vi "DAQ_DC-RMS Voltage Meas Initialize.vi"(0 "Physical Channels":tag, 7 "Global Channels":refnum<k21>, 11 "error in":errorcluster) -> (4 "DAQmx Task Out":refnum<k21>, 15 "error out":errorcluster)   [LabVIEW 2021, in "DAQ_DC-RMS Voltage Measurement.lvlib"]
doc: "Initialize analog input channels and obtains a DAQmx task\n\nProvide either Physical channel or Global Channel\nIf both physical and Global channels are provided, Global Channels will take precedence"
uses:
  DAQ_DC-RMS Voltage Measurement.lvlib
  <vilib>/DAQmx/create/channels.llb/DAQmx Create Channel (AI-Voltage-Basic).vi
panel:
  # "Inputs"
  # "Outputs"
  # "Overview:\nThis VI interacts with the DAQ driver to initialize an instrument and provide a corresponding instrument handle\n\nHardware Requirements: A compatible PXI, PCIe, USB, cDAQ or Testscale device\n\nSoftware Requirements: NI DAQmx 2022 Q4 or later\n\nInstructions:\n1. Enter physical channel in which DC Voltage Measurement has to be done in Physical Channels control. (Or) Enter Global channels to use it instead of initiating a new task. User must configure only one input. If both are provided, Global Channels will take precedence.\n3. Get the DC Voltage Measurement task from DAQmx Task Out\n\nNote: User can use the DAQmx Task on other APIs to configure and initiate DC-RMS Voltage and Measurements."
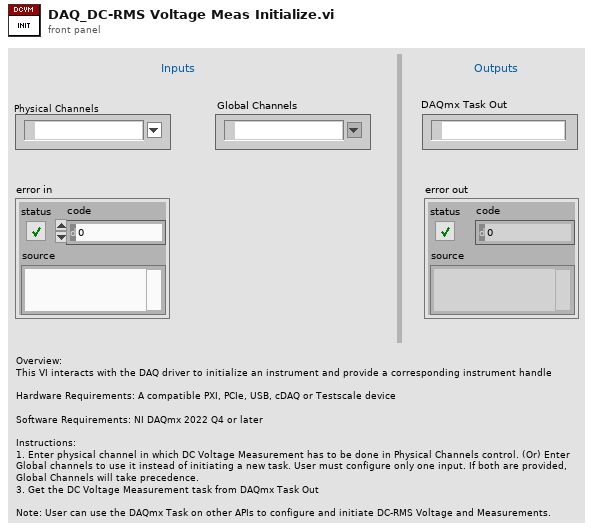
[diagram p1: front panel]
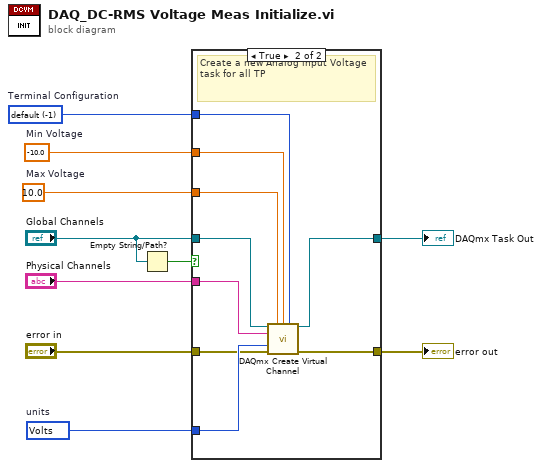
[diagram p0: block diagram]
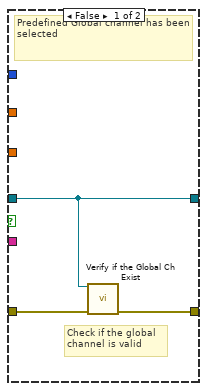
[diagram p2: hidden frame]
diagram:
  w3 = -1 items=["default"=-1, "RSE"=10083, "NRSE"=10078, "Differential"=10106, "Pseudodifferential"=12529]  # Terminal Configuration
  w4 = -10.0  # Min Voltage
  w5 = 10.0  # Max Voltage
  w10 = 10348 items=["Volts"=10348, "From Custom Scale"=10065]  # units
  n1 = Empty String/Path?(string/path="Global Channels") -> (empty?=w2:bool)
  n2 = case shown="True" w2 {
    tunnel: "Physical Channels" -> [_ w18]
    tunnel: "Global Channels" -> [w11 w22]
    tunnel: [w11 w21] -> w6
    tunnel: "error in" -> [w13 w19]
    tunnel: [w12 w17] -> w9
    tunnel: w10 -> [_ w20]
    tunnel: w5 -> [_ w16]
    tunnel: w4 -> [_ w15]
    tunnel: w3 -> [_ w14]
    frame False {
      # "Check if the global\nchannel is valid"
      # "Predefined Global channel has been selected"
      n3 = call "Verify if the Global Ch Exist.vi"("Global Channels"=w11, "error in (no error)"=w13) -> ("error out"=w12:errorcluster)  [unwired: 13 in]
    }
    frame True {
      # "Create a new Analog input Voltage task for all TP"
      n4 = call-poly <vilib>:"DAQmx Create Virtual Channel.vi"("task in"=w22, "maximum value"=w16, "minimum value"=w15, "input terminal configuration"=w14, "physical channels"=w18, "units"=w20, "error in"=w19) -> ("task out"=w21:refnum<k21>, "error out"=w17:errorcluster)  [unwired: 7 in]
    }
  }
  "DAQmx Task Out" <- w6
  "error out" <- w9
